vi "get_config_cluster.vi"(8 "error in (no error)":errorcluster, 11 "GenericPlugin in":refnum<class "StageMMS2015ASI.lvclass">) -> (0 "error out":errorcluster, 2 "config cluster (variant)":variant, 3 "GenericPlugin out":refnum<class "StageMMS2015ASI.lvclass">)   [LabVIEW 2010, in "StageMMS2015ASI.lvclass"]
uses:
  StageMMS2015ASI.lvclass
  StageMMS2015ASI.lvclass/StageMMS2015ASI.ctl
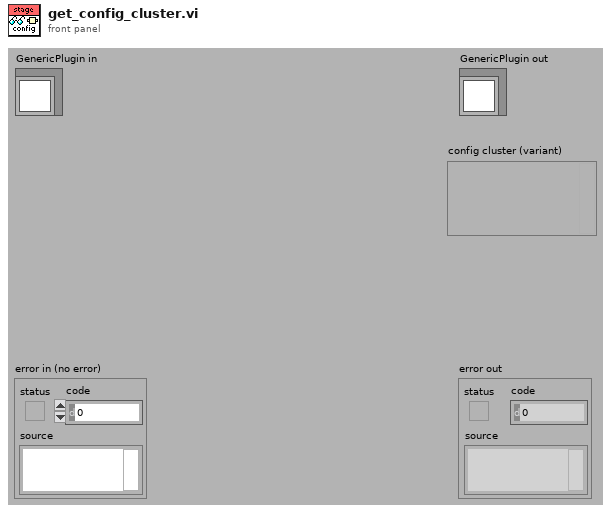
[diagram p1: front panel]
types:
  T1 = typedef "StageMMS2015ASI.lvclass/config_data_cluster.ctl" = cluster{"serial port":string, "speed":dbl[unit], "step factor":dbl[unit]}
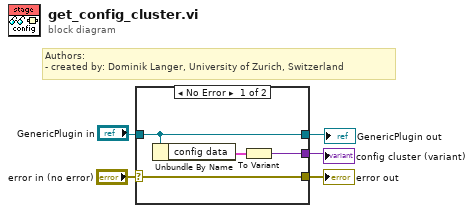
[diagram p0: block diagram]
diagram:
  # "Authors: \n- created by: Dominik Langer, University of Zurich, Switzerland"
  n1 = case shown="No Error" "error in (no error)" {
    selector: "error in (no error)" -> [w9 w10]
    tunnel: "GenericPlugin in" -> [w8 w11]
    tunnel: [w9 w10] -> w1
    tunnel: [w8 w11] -> w3
    tunnel: [w6 _] -> w2
    frame No Error {
      n2 = Unbundle By Name(w8) -> ("config data"=w7:T1)
      n3 = To Variant(anything=w7) -> (Variant=w6:variant)
    }
    frame Error {
    }
  }
  "error out" <- w1
  "GenericPlugin out" <- w3
  "config cluster (variant)" <- w2
